vi "Intake Teleop.vi"(11 "Axes":dbl[](array[numeric])) -> ()   [LabVIEW 2020]
uses:
  Types/Axes.ctl
  67a21d00-8447-4962-960d-252d432a3f8b.vi
panel:
  in  "Intake Power":dbl=0.5
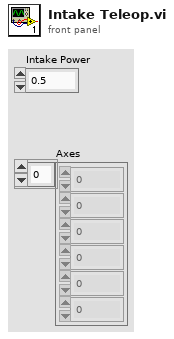
[diagram p1: front panel]
types:
  T1 = typedef "Axes.ctl" = enum16{"LX", "LY", "LT", "RT", "RX", "RY"}
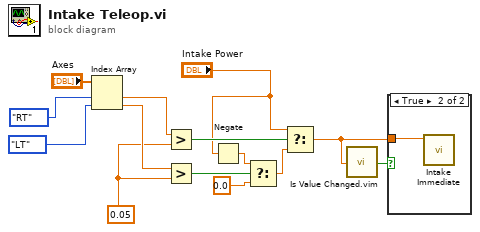
[diagram p0: block diagram]
diagram:
  w7 = 0.05 ("y")
  n1 = Index Array(array="Axes", index #1=Axes."RT" ("Axes"), index #2=Axes."LT" ("Axes")) -> (element #1=w5:dbl, element #2=w11:dbl)
  n2 = Greater?(x=w5, y=w7) -> (0:w6:bool)
  n3 = Greater?(x=w11, y=w7) -> (0:w12:bool)
  n4 = Negate(x="Intake Power") -> (-x=w10:dbl)
  n5 = Select(t=w10, s=w12, f=0.0) -> (s? t:f=w8:dbl)
  n6 = Select(t="Intake Power", s=w6, f=w8) -> (s? t:f=w2:dbl)
  n7 = call "Is Value Changed.vim"("value"=w2) -> ("changed or first call?"=w1:bool)
  n8 = case shown="True" w1 {
    tunnel: w2 -> [_ w15]
    frame False {
    }
    frame True {
      n9 = call "Intake Immediate.vi"("Setpoint"=w15) -> ()  [unwired: 10 in, 1 out]
    }
  }
